vi "BasicExampleOCP.vi"() -> ()   [LabVIEW 2025]
uses:
  PalmSens/PalmSens.lvclass
  PalmSens/MeasurementResults.ctl
  PalmSens/LiveCurveResult.ctl
  E:/PSCode/PalmSens_SDK/labview/PalmSens/Libraries/PalmSens.Core.Simplified.LabVIEW.dll
  PalmSens/Libraries/PalmSens.Core.Simplified.LabVIEW.dll
panel:
  out "Method Indicator":refnum<k24>
  out "Curves":T1
  out "Array":string[](array[string])
  out "Is Measuring":bool
  in  "PalmSens.lvclass":refnum<class "PalmSens.lvclass">
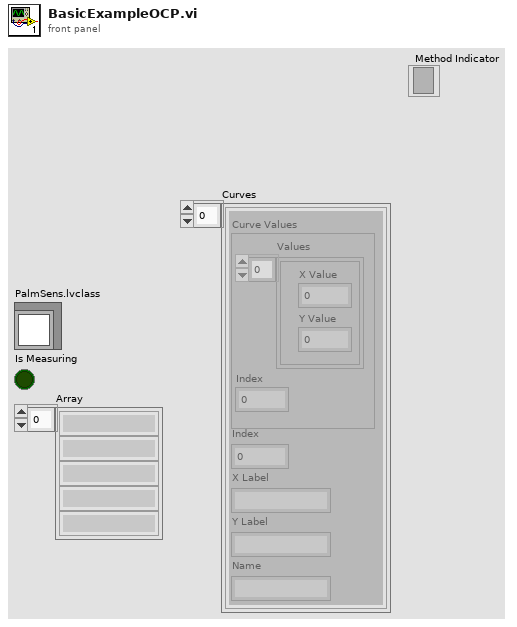
[diagram p1: front panel]
types:
  T1 = typedef "MeasurementResults.ctl" = T2[]
  T2 = typedef "LiveCurveResult.ctl" = cluster{"X Label":string, "Y Label":string, "Name":string, "Index":i16, "Curve Values":cluster{"Values":cluster{"X Value":dbl, "Y Value":dbl}[], "Index":i16}}
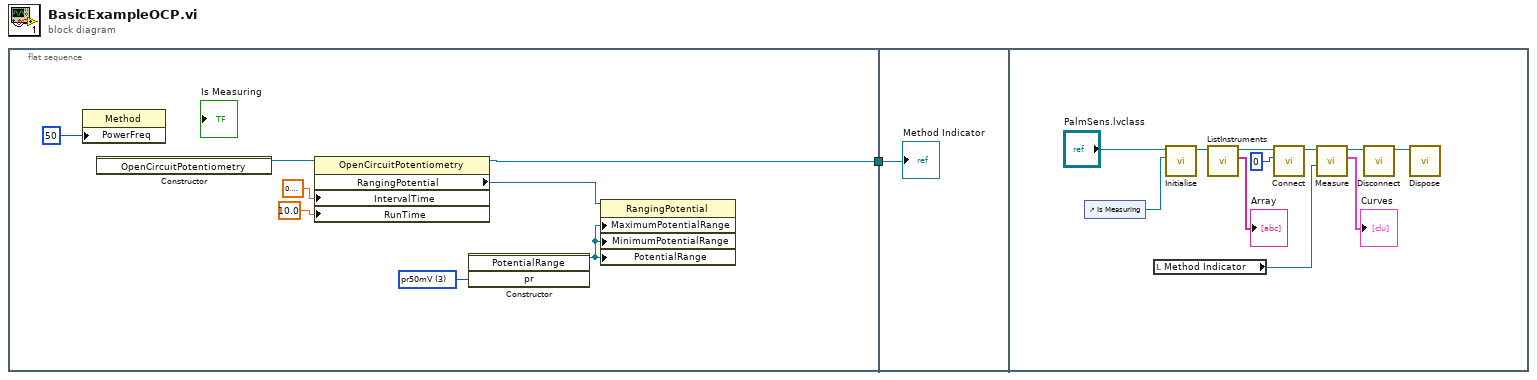
[diagram p0: block diagram]
diagram:
  n1 = flat-sequence {
    tunnel: [w2] -> w1
    tunnel: w1 -> [w10]
    frame #0 {
      w6 = 3 items=["pr1mV", "pr10mV", "pr20mV", "pr50mV", "pr100mV", "pr200mV", "pr500mV", "pr1V"] ("pr")
      n2 = property class="Method"("PowerFreq"=50) -> ()  [unwired: 2 in, 2 out]
      n3 = constructor class="OpenCircuitPotentiometry"() -> (reference out=w7:refnum<k24>)  [unwired: 3 in, 2 out]
      n4 = property class="OpenCircuitPotentiometry"(reference=w7, "IntervalTime"=sgl 0.1, "RunTime"=sgl 10.0) -> (reference out=w2:refnum<k24>, "RangingPotential"=w8:refnum<k24>)  [unwired: 1 in, 1 out]
      n5 = constructor class="PotentialRange"("pr"=w6) -> (reference out=w9:refnum<k24>)  [unwired: 3 in, 3 out]
      n6 = property class="RangingPotential"(reference=w8, "MaximumPotentialRange"=w9, "MinimumPotentialRange"=w9, "PotentialRange"=w9) -> ()  [unwired: 1 in, 2 out]
    }
    frame #1 {
      "Method Indicator" <- w10
    }
    frame #2 {
      n7 = control-ref of="Is Measuring"() -> (w13:refnum<vi>)
      n8 = local read "Method Indicator"() -> (w21:refnum<k24>)
      n9 = call-dynamic "Initialise.vi"("Is Measuring Refnum"=w13, "PalmSens in"="PalmSens.lvclass") -> ("PalmSens out"=w14:refnum<class "PalmSens.lvclass">)  [unwired: 8 in, 1 out]
      n10 = call-dynamic "ListInstruments.vi"("PalmSens in"=w14) -> ("Array"=→"Array":string[], "PalmSens out"=w16:refnum<class "PalmSens.lvclass">)  [unwired: 8 in, 1 out]
      n11 = call-dynamic "Connect.vi"("Instrument Index"=0, "PalmSens in"=w16) -> ("PalmSens out"=w19:refnum<class "PalmSens.lvclass">)  [unwired: 8 in, 1 out]
      n12 = call-dynamic "Measure.vi"("Method .NET Refnum"=w21, "PalmSens in"=w19) -> ("Curves"=→"Curves":T1, "PalmSens out"=w18:refnum<class "PalmSens.lvclass">)  [unwired: 2 in, 2 out]
      n13 = call-dynamic "Disconnect.vi"("PalmSens in"=w18) -> ("PalmSens out"=w17:refnum<class "PalmSens.lvclass">)  [unwired: 9 in, 1 out]
      n14 = call-dynamic "Dispose.vi"("PalmSens in"=w17) -> ()  [unwired: 9 in, 2 out]
    }
  }
